vi "configCNT.vi"(8 "error in (no error)":errorcluster, 10 "Channel  1":i32(ring) items=["A", "B"]) -> (0 "error out":errorcluster)   [LabVIEW 2019, in "CNT90_GPIB.lvlib"]
uses:
  CNT90_GPIB.lvlib
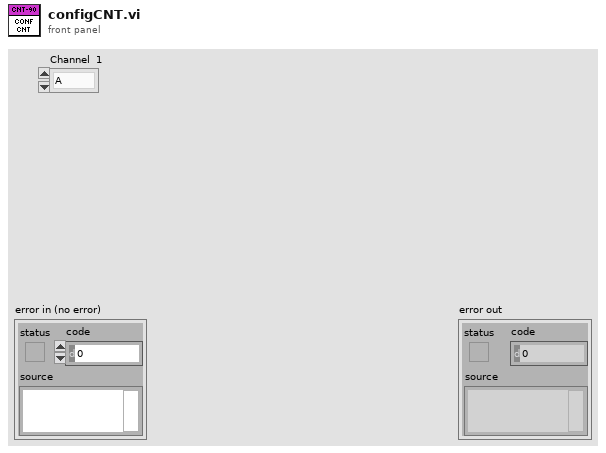
[diagram p1: front panel]
types:
  T1 = cluster{"error":bool, "code":i32, "source":string}
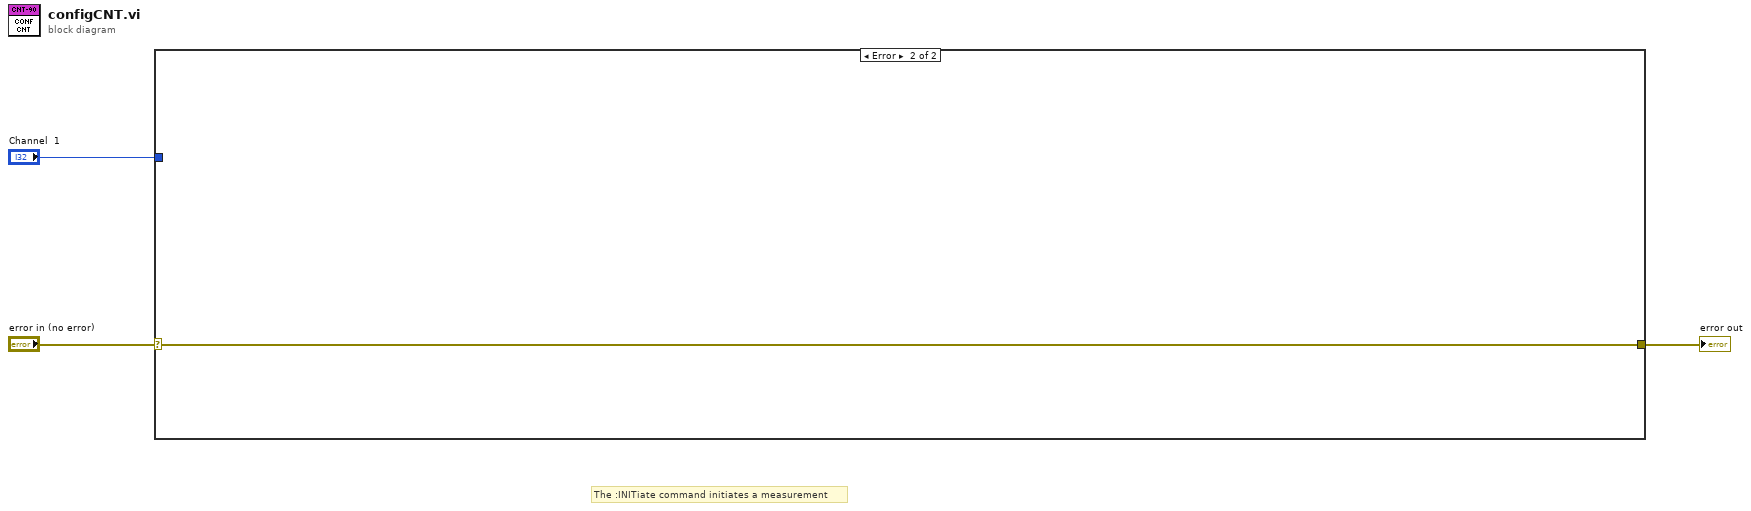
[diagram p0: block diagram]
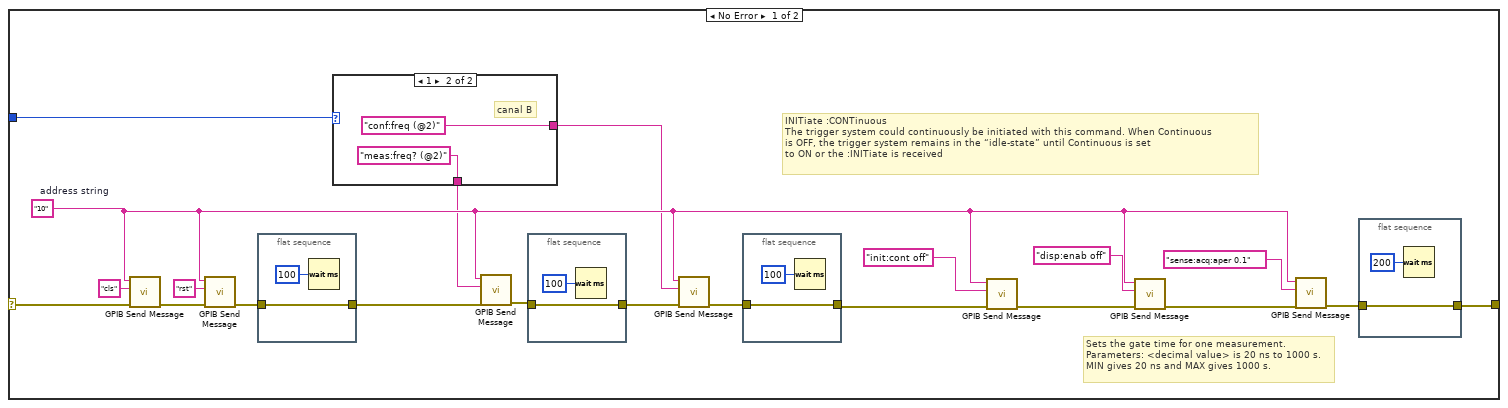
[diagram p2: hidden frame]
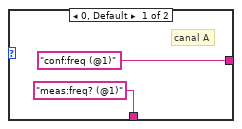
[diagram p3: hidden frame]
diagram:
  # "The :INITiate command initiates a measurement"
  n1 = case shown="Error" "error in (no error)" {
    selector: "error in (no error)" -> [w8 w37]
    tunnel: [w7 w37] -> w2
    tunnel: "Channel  1" -> [w6 _]
    frame No Error {
      w14 = "10"  # address string
      # "Sets the gate time for one measurement.\nParameters: <decimal value> is 20 ns to 1000 s.\nMIN gives 20 ns and MAX gives 1000 s."
      # "INITiate :CONTinuous\nThe trigger system could continuously be initiated with this command. When Continuous\nis OFF, the trigger system remains in the “idle-state” until Continuous is set\nto ON or the :INITiate is received"
      n2 = call <instrlib>:"GPIB Send Message.vi"("address string"=w14, "write buffer"="cls", "error in"=w8) -> ("error out"=w22:T1)  [unwired: 4 in, 2 out]
      n3 = call <instrlib>:"GPIB Send Message.vi"("address string"=w14, "write buffer"="rst", "error in"=w22) -> ("error out"=w20:T1)  [unwired: 4 in, 2 out]
      n4 = flat-sequence {
        tunnel: [w34] -> w21
        tunnel: w20 -> [w34]
        frame #0 {
          n5 = Wait (ms)(milliseconds to wait=u32 100) -> ()  [unwired: 1 out]
        }
      }
      n6 = case shown="1" w6 {
        tunnel: ["conf:freq (@1)" ("write buffer") "conf:freq (@2)" ("write buffer")] -> w5
        tunnel: ["meas:freq? (@1)" ("write buffer") "meas:freq? (@2)" ("write buffer")] -> w4
        frame 0, Default {
          # "canal A"
        }
        frame 1 {
          # "canal B"
        }
      }
      n7 = call <instrlib>:"GPIB Send Message.vi"("address string"=w14, "write buffer"=w4, "error in"=w21) -> ("error out"=w19:T1)  [unwired: 4 in, 2 out]
      n8 = flat-sequence {
        tunnel: [w32] -> w18
        tunnel: w19 -> [w32]
        frame #0 {
          n9 = Wait (ms)(milliseconds to wait=u32 100) -> ()  [unwired: 1 out]
        }
      }
      n10 = call <instrlib>:"GPIB Send Message.vi"("address string"=w14, "write buffer"=w5, "error in"=w18) -> ("error out"=w17:T1)  [unwired: 4 in, 2 out]
      n11 = flat-sequence {
        tunnel: [w30] -> w16
        tunnel: w17 -> [w30]
        frame #0 {
          n12 = Wait (ms)(milliseconds to wait=u32 100) -> ()  [unwired: 1 out]
        }
      }
      n13 = call <instrlib>:"GPIB Send Message.vi"("address string"=w14, "write buffer"="init:cont off", "error in"=w16) -> ("error out"=w15:T1)  [unwired: 4 in, 2 out]
      n14 = call <instrlib>:"GPIB Send Message.vi"("address string"=w14, "write buffer"="disp:enab off", "error in"=w15) -> ("error out"=w24:T1)  [unwired: 4 in, 2 out]
      n15 = call <instrlib>:"GPIB Send Message.vi"("address string"=w14, "write buffer"="sense:acq:aper 0.1", "error in"=w24) -> ("error out"=w23:T1)  [unwired: 4 in, 2 out]
      n16 = flat-sequence {
        tunnel: [w36] -> w7
        tunnel: w23 -> [w36]
        frame #0 {
          n17 = Wait (ms)(milliseconds to wait=u32 200) -> ()  [unwired: 1 out]
        }
      }
    }
    frame Error {
    }
  }
  "error out" <- w2
